vi "Write Sweep configuration.vi"(8 "error in (no error)":errorcluster, 10 "Configuration":T1 {"Sweep  rate" format="%#_6p"; "End sweep" format="%#_6p"; "Start sweep" format="%#_6p"}, 11 "Sweeper  in":refnum<class "Sweeper.lvclass">) -> (0 "error out":errorcluster, 3 "Sweeper  out":refnum<class "Sweeper.lvclass">)   [LabVIEW 2016, in "Sweeper.lvclass"]
uses:
  Sweeper.lvclass
  C:/github/LabActor/Template Module/Template Module.lvclass
  NHMFL_Core/Libraries/Instruments/Instrument Driver/Sweeper Driver/Sweep Configuration.ctl
  Template Module/Template Module.lvclass/Template Module.ctl
  Template Module/Write Configuration.vi
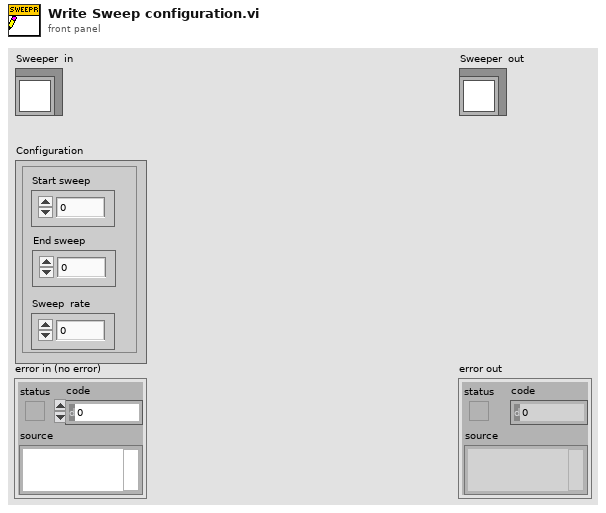
[diagram p1: front panel]
types:
  T1 = typedef "Sweep Configuration.ctl" = cluster{"Start sweep":dbl, "End sweep":dbl, "Sweep  rate":dbl}
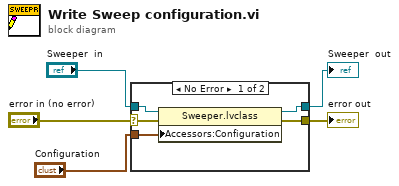
[diagram p0: block diagram]
diagram:
  n1 = case shown="No Error" "error in (no error)" {
    selector: "error in (no error)" -> [w8 w11]
    tunnel: [w7 w11] -> w4
    tunnel: [w6 w12] -> w2
    tunnel: "Sweeper  in" -> [w10 w12]
    tunnel: "Configuration" -> [w9 _]
    frame No Error {
      n2 = property class="Sweeper.lvclass"(reference=w10, error in=w8, "Accessors:Configuration"=w9) -> (reference out=w6:refnum<class "Sweeper.lvclass">, error out=w7:errorcluster)
    }
    frame Error {
    }
  }
  "error out" <- w4
  "Sweeper  out" <- w2
